vi "set_report_class.vi"(7 "error in (no error)":errorcluster, 10 "UI_out in":T1) -> (0 "error out":errorcluster, 3 "UI_out out":T1)   [LabVIEW 2017]
uses:
  ui.ctl
  classes/dc_power_supply/DC_power_supply.lvclass
  classes/report/Report.lvclass
  ui_buttons.ctl
  types/boc_type.ctl
  classes/report/excel/boc6/Boc6.lvclass
  classes/report/excel/boc12/Boc12.lvclass
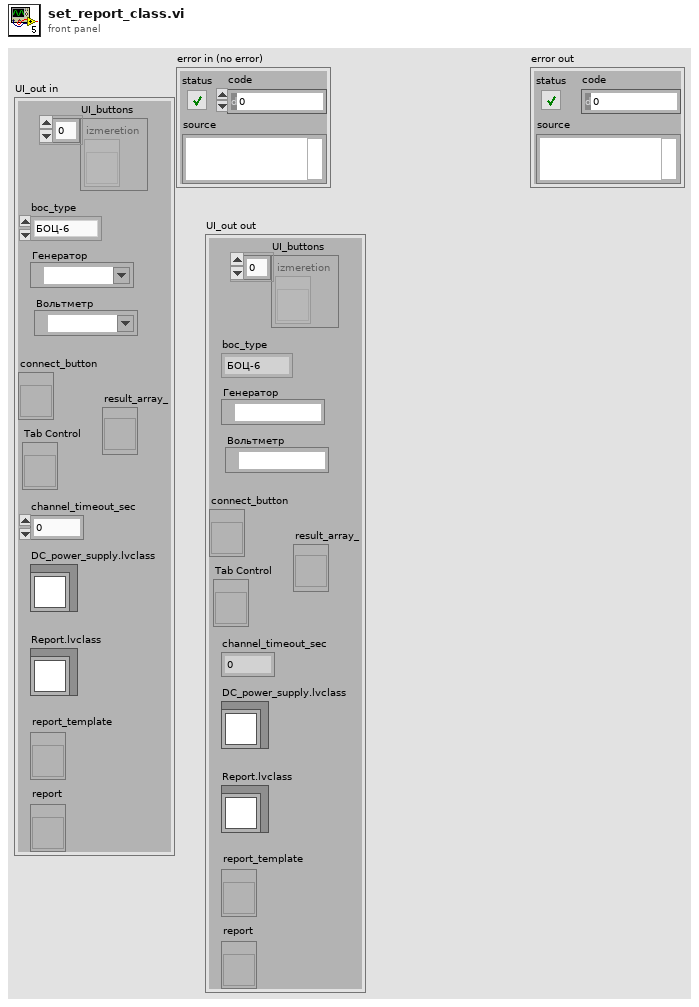
[diagram p1: front panel]
types:
  T1 = typedef "ui.ctl" = cluster{"UI_buttons":T2, "Tab Control":refnum<vi>, "connect_button":refnum<vi>, "generator":refnum<visa-resource-name>, "voltmetr":refnum<visa-resource-name>, "channel_timeout_sec":dbl, "boc_type":T3, "result_array_":refnum<vi>, "DC_power_supply.lvclass":refnum<class "DC_power_supply.lvclass">, "Report.lvclass":refnum<class "Report.lvclass">, "report_template":refnum<vi>, "report":refnum<vi>}
  T2 = typedef "ui_buttons.ctl" = refnum<vi>[]
  T3 = typedef "boc_type.ctl" = enum16{"БОЦ-6", "БОЦ-12"}
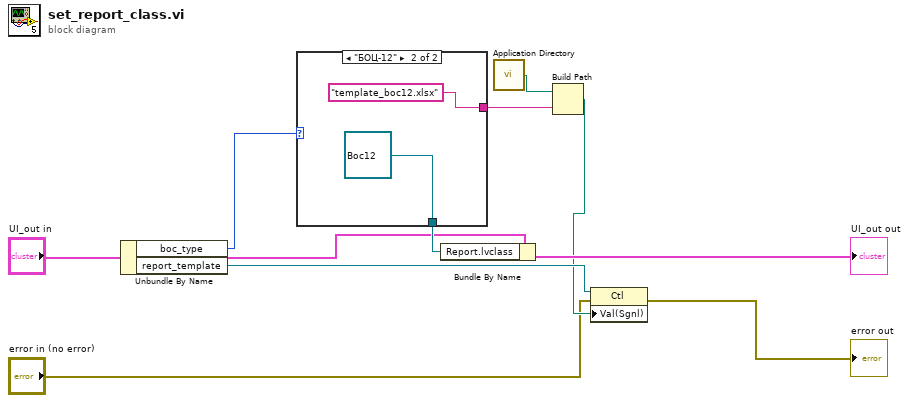
[diagram p0: block diagram]
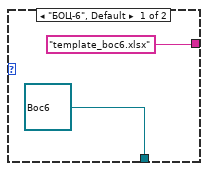
[diagram p2: hidden frame]
diagram:
  n1 = Unbundle By Name("UI_out in") -> ("boc_type"=w3:T3, "report_template"=w6:refnum<vi>)
  n2 = case shown="\"БОЦ-12\"" w3 {
    tunnel: [refnum<class "Boc6.lvclass"> refnum ("Boc6.lvclass") refnum<class "Boc12.lvclass"> refnum ("Boc12.lvclass")] -> w9
    tunnel: ["template_boc6.xlsx" ("name or relative path") "template_boc12.xlsx" ("name or relative path")] -> w7
    frame "БОЦ-6", Default {
    }
    frame "БОЦ-12" {
    }
  }
  n3 = Bundle By Name(cluster="UI_out in", "Report.lvclass"=w9) -> (→"UI_out out":T1)
  n4 = call <vilib>:"Application Directory.vi"() -> ("Application Directory"=w4:path)
  n5 = Build Path(base path=w4, name or relative path=w7) -> (appended path=w5:path)
  n6 = property class="Ctl"(reference=w6, error in="error in (no error)", "Val(Sgnl)"=w5) -> (error out=→"error out":errorcluster)  [unwired: 1 out]
